vi "DebugInit.vi"(8 "errin":errorcluster, 10 "debug?":bool, 11 "VISA Refnum in":refnum<visa-resource-name>) -> (0 "error out":errorcluster, 1 "OF":string, 2 "queue out":refnum<queue>)   [LabVIEW 2020]
uses:
  VarGLO/Global PEAK.vi
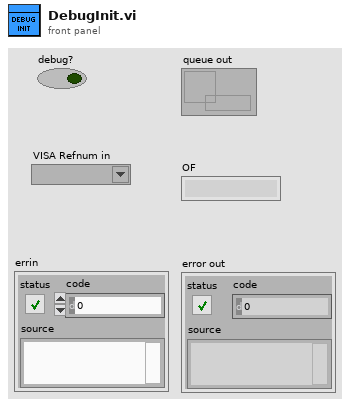
[diagram p1: front panel]
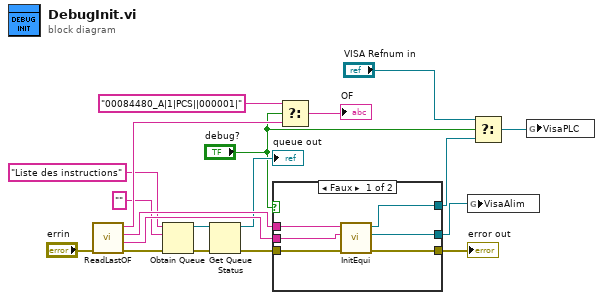
[diagram p0: block diagram]
diagram:
  n1 = call "ReadLastOF.vi"("errin"="errin") -> ("errout"=w9:errorcluster, "VISA HITECH"=w11:string, "VISA Auto"=w10:string, "OF"=w12:string)  [unwired: 7 in]
  n2 = Obtain Queue ("Obtenir une file d'attente")(name (unnamed)="Liste des instructions" ("nom (aucun)"), element data type="", error in (no error)=w9) -> (queue out=w6:refnum<queue>, error out=w7:errorcluster)  [unwired: 2 in, 1 out]
  n3 = Get Queue Status ("Obtenir l'état d'une file d'attente")(queue=w6, error in (no error)=w7) -> (queue out=→"queue out":refnum<queue>, error out=w16:errorcluster)  [unwired: 1 in, 6 out]
  n4 = case shown="Faux" "debug?" {
    tunnel: [w25 _] -> w19
    tunnel: [w24 w26] -> w17
    tunnel: w16 -> [w23 w26]
    tunnel: w11 -> [w22 _]
    tunnel: w10 -> [w21 _]
    tunnel: [w20 _] -> w1
    frame False {
      n5 = call "InitEqui.vi"("errin"=w23, "VISA HITECH"=w22, "VISA Auto"=w21) -> ("errout"=w24:errorcluster, "VisaHitech"=w20:refnum<visa-resource-name>, "VISA Refnum out"=w25:refnum<visa-resource-name>)  [unwired: 6 in]
    }
    frame True {
    }
  }
  "error out" <- w17
  n6 = Select(t="00084480_A|1|PCS||000001|" ("OFnext"), s="debug?", f=w12) -> (s? t:f=→"OF":string)
  n7 = global write "Global PEAK.vi" "VisaAlim"(w1) -> ()
  n8 = Select(t="VISA Refnum in", s="debug?", f=w19) -> (s? t:f=w3:refnum<visa-resource-name>)
  n9 = global write "Global PEAK.vi" "VisaPLC"(w3) -> ()
